vi "AddControlCompane__slk_mt.vi"(8 "error in (no error)":errorcluster, 10 "vi name":string, 11 "application reference":refnum<vi>) -> (0 "error out":errorcluster)   [LabVIEW 2015, in "Lazyboots Menu Tool.lvlib"]
uses:
  <vilib>/SLK/Lazyboots Menu Tool/Library/Lazyboots Menu Tool.lvlib
  <vilib>/SLK/Lazyboots Menu Tool/Private/AddControlConpane/TydeDef/TypeDef_AddControlConpane__slk_mt.ctl
  <vilib>/Utility/config.llb/NI_LVConfig.lvlib
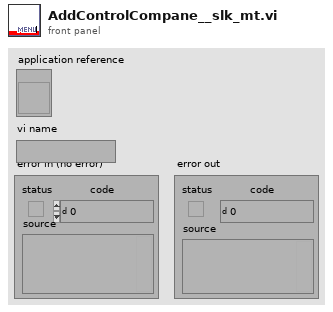
[diagram p1: front panel]
types:
  T1 = typedef "Lazyboots Menu Tool.lvlib/TypeDef_AddControlConpane__slk_mt.ctl" = enum16{"Read Configure", "Get Menu Launch VI", "Undo.Start", "Add Control Conpane", "Undo.End/Fail", "End"}
  T2 = typedef "NI_LVConfig.lvlib/Config Data RefNum.ctl" = refnum<k1>
  T3 = typedef "Lazyboots Menu Tool.lvlib/TypeDef_AddErrorCaseConfigure__slk_mt.ctl" = cluster{"Frame Width":u32, "Create Constant":bool}
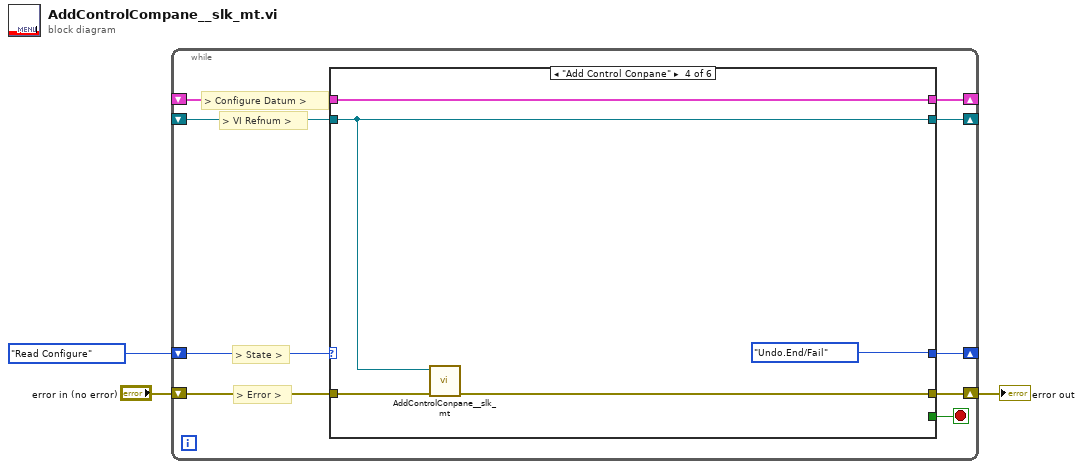
[diagram p0: block diagram]
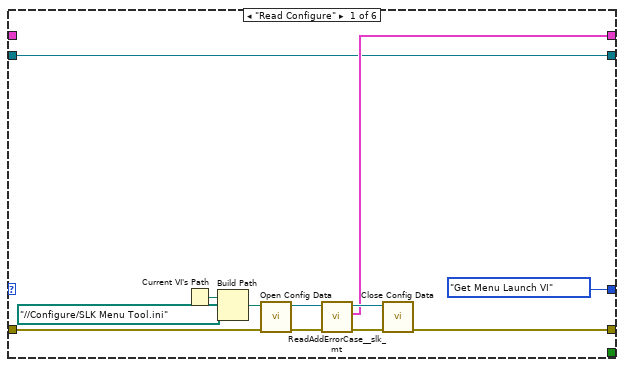
[diagram p2: hidden frame]
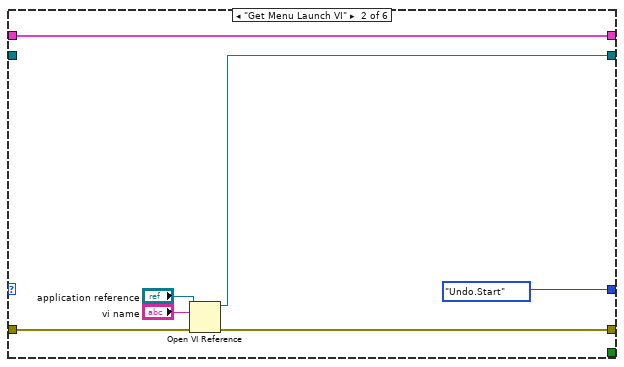
[diagram p3: hidden frame]
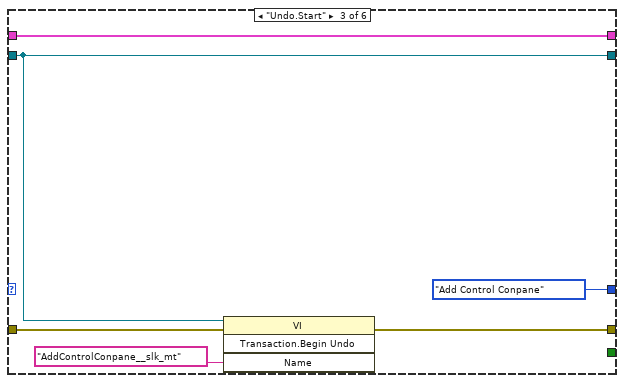
[diagram p4: hidden frame]
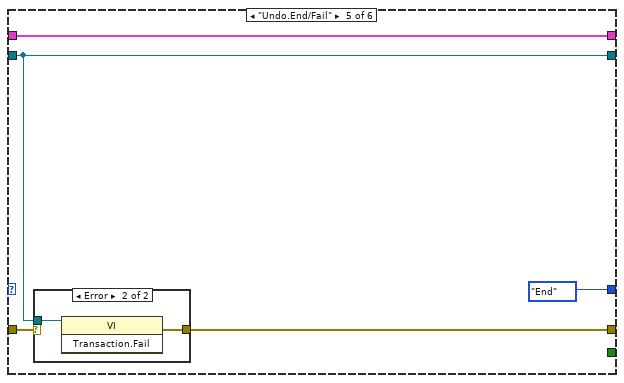
[diagram p5: hidden frame]
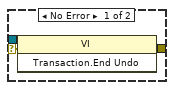
[diagram p6: hidden frame]
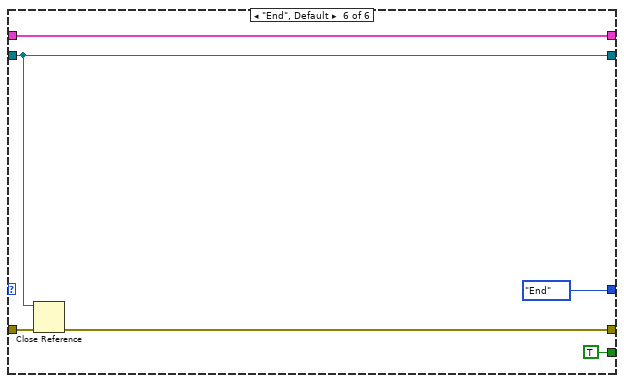
[diagram p7: hidden frame]
diagram:
  n1 = while {
    shift-right: [w9] -> _
    shift-left: TypeDef_AddControlConpane__slk_mt."Read Configure" ("State") -> [w12]
    shift-right: [w10] -> w2
    shift-left: "error in (no error)" -> [w11]
    shift-right: [w7] -> _
    shift-left: _ -> [w8]
    shift-right: [w5] -> _
    shift-left: _ -> [w6]
    stop <- w4 stop-if-true
    # "> VI Refnum >"
    # "> Configure Datum >"
    # "> Error >"
    # "> State >"
    n2 = case shown="\"Add Control Conpane\"" w12 {
      tunnel: w11 -> [w18 w31 w36 w39 w46 w54]
      tunnel: [w16 w29 w35 w38 w45 w56] -> w10
      tunnel: [TypeDef_AddControlConpane__slk_mt."Get Menu Launch VI" ("State") TypeDef_AddControlConpane__slk_mt."Undo.Start" ("State") TypeDef_AddControlConpane__slk_mt."Add Control Conpane" ("State") TypeDef_AddControlConpane__slk_mt."Undo.End/Fail" ("State") TypeDef_AddControlConpane__slk_mt."End" ("State") TypeDef_AddControlConpane__slk_mt."End" ("State")] -> w9
      tunnel: w8 -> [_ w28 w37 w42 w47 w58]
      tunnel: [w15 w28 w37 w42 w47 w58] -> w7
      tunnel: w6 -> [w14 _ w34 w40 w44 w55]
      tunnel: [w14 w27 w34 w40 w44 w55] -> w5
      tunnel: [_ _ _ _ _ TRUE] -> w4
      frame "Read Configure" {
        n3 = Current VI's Path() -> (path=w20:path)
        n4 = Build Path(base path=w20, name or relative path=path "../../Configure/SLK Menu Tool.ini") -> (appended path=w19:path)
        n5 = call <vilib>:"Open Config Data.vi"("error in (no error)"=w18, "configuration file path"=w19) -> ("error out"=w23:errorcluster, "refnum"=w24:T2)  [unwired: 7 in, 1 out]
        n6 = call <vilib>:"ReadAddErrorCase__slk_mt.vi"("error in (no error)"=w23, "refnum in"=w24) -> ("error out"=w22:errorcluster, "add error case configure"=w15:T3, "refnum out"=w21:T2)  [unwired: 7 in]
        n7 = call <vilib>:"Close Config Data.vi"("error in (no error)"=w22, "refnum"=w21) -> ("error out"=w16:errorcluster)  [unwired: 8 in, 1 out]
      }
      frame "Get Menu Launch VI" {
        n8 = Open VI Reference(application reference (local)="application reference", vi path="vi name", error in (no error)=w31) -> (vi reference=w27:refnum<vi>, error out=w29:errorcluster)  [unwired: 3 out]
      }
      frame "Undo.Start" {
        n9 = invoke class="VI" method="Transaction.Begin Undo"(reference=w34, error in=w36, "Name"="AddControlConpane__slk_mt") -> (error out=w35:errorcluster)  [unwired: 1 in, 3 out]
      }
      frame "Add Control Conpane" {
        n10 = call <vilib>:"AddControlConpane__slk_mt.vi"("error in (no error)"=w39, "This VI"=w40) -> ("error IO"=w38:errorcluster)  [unwired: 9 in]
      }
      frame "Undo.End/Fail" {
        n11 = case shown="Error" w46 {
          selector: w46 -> [w49 _]
          tunnel: w44 -> [w50 w52]
          tunnel: [w48 w51] -> w45
          frame No Error {
            n12 = invoke class="VI" method="Transaction.End Undo"(reference=w50, error in=w49) -> (error out=w48:errorcluster)  [unwired: 1 in, 2 out]
          }
          frame Error {
            n13 = invoke class="VI" method="Transaction.Fail"(reference=w52) -> (error out=w51:errorcluster)  [unwired: 2 in, 2 out]
          }
        }
      }
      frame "End", Default {
        n14 = Close Reference(reference=w55, error in (no error)=w54) -> (error out=w56:errorcluster)
      }
    }
  }
  "error out" <- w2
